vi "RTS Relay Status.vi"(0 "Chamber 1 Socket":string[][](array[string]), 1 "Tree Selection":T1="Select Room/Stall", 5 "Chamber 2 Socket":string[][](array[string]), 7 "Chamber 3 Socket":string[][](array[string]), 9 "Chamber 4 Socket":string[][](array[string]), 11 "error in (no error)":errorcluster, 12 "Extract Column":i32=73) -> (2 "Station 1":i32, 3 "Station 2":i32, 4 "Station 3":i32, 6 "Station 4":i32, 8 "Station 5":i32, 10 "Station 6":i32, 13 "Station 8":i32, 14 "Station 7":i32, 15 "error out":errorcluster)   [LabVIEW 2016]
uses:
  Type Definitions/RTS Room Selector.ctl
panel:
  in  "Debug":string[][](array[string])=[["System Date", "System Time", "Elapsed Time (sec)", "Elapsed Time (hrs)", "Voltage (V)", "RMS Current (Amps)", "Power (Watts)", "Watt Hours (Wh)", "Voltage Total Harmonic Distortion (%)", "Frequency (Hz)", "Apparent Power (VA)", "Power Factor", "TC 1", "TC 2", "TC 3", "TC 4", "TC 5", "TC 6", "TC 7", "TC 8", "TC 9", "TC 10", "TC 11", "TC 12", "TC 13", "TC 14", "TC 15", "TC 16", "TC 17", "TC 18", "TC 19", "TC 20", "TC 21", "TC 22", "TC 23", "TC 24", "TC 25", "TC 26", "TC 27", "TC 28", "TC 29", "TC 30", "AUX 1", "AUX 2", "CAL CL", "Room Setpoint Temperature", "Room Setpoint Humidity", "Room Temperature (°F)", "Room Humidity (%)", "Door Enable", "Room Setpoint Cool Temperature", "Room Setpoint Dehumidification Temperature", "Supply Temperature (°F)", "Cool Temperature (°F)", "Dehumidification Temperature (°F)", "Glycol Temperature (°F)", "Heat Rate (%)", "Steam Rate (%)", "Cool Rate (%)", "Dehumidification Rate (%)", "Room Status", "Room Dry P", "Room Dry I", "Room Humidity P", "Room Humidity I", "Room Heat P", "Room Heat I", "Room Cool Temperature P", "Room Cool Temperature I", "Room Dehumidification Temperature P", "Room Dehumidification Temperature I", "Voltage Setpoint 1", "60 Hz Power", "50 Hz Power", "120V Range", "240V Range", "Ground Line", "Ground Neutral", "Measure Ground Leakage Current", "Room OK", "S1 Freezer Relay", "S1 Cab Relay", "S1 Slide Relay", "Recording Data", "CVS Location", "Point Location"], ["01/23/2018", "08:26:39.773", "0.000000", "0.000000", "119.742401", "0.732354", "75.278603", "510.887438", "3.300000", "59.994091", "87.224380", "0.863045", "8.350000", "8.210000", "10.270000", "327.670000", "327.670000", "327.670000", "327.670000", "327.670000", "327.670000", "327.670000", "37.750000", "35.520000", "35.220000", "327.670000", "327.670000", "327.670000", "327.670000", "327.670000", "327.670000", "327.670000", "327.670000", "327.670000", "327.670000", "70.660000", "327.670000", "327.670000", "70.440000", "327.670000", "32767.000000", "32767.000000", "0.001000", "0.000000", "1.988000", "70.000000", "35.000000", "69.850000", "38.830000", "1.000000", "55.000000", "48.000000", "67.060000", "55.180000", "48.160000", "0.000000", "38.280000", "0.000000", "30.610000", "8.190000", "0.000000", "200.000000", "15000.000000", "400.000000", "15000.000000", "1000.000000", "2000.000000", "500.000000", "6000.000000", "500.000000", "6000.000000", "120.000000", "1.000000", "0.000000", "1.000000", "0.000000", "0", "1.000000", "0.000000", "0.000000", "0.000000", "0.000000", "0.000000", "FALSE", "", ""], ["System Date", "System Time", "Elapsed Time (sec)", "Elapsed Time (hrs)", "Voltage (V)", "RMS Current (Amps)", "Power (Watts)", "Watt Hours (Wh)", "Voltage Total Harmonic Distortion (%)", "Frequency (Hz)", "Apparent Power (VA)", "Power Factor", "TC 1", "TC 2", "TC 3", "TC 4", "TC 5", "TC 6", "TC 7", "TC 8", "TC 9", "TC 10", "TC 11", "TC 12", "TC 13", "TC 14", "TC 15", "TC 16", "TC 17", "TC 18", "TC 19", "TC 20", "TC 21", "TC 22", "TC 23", "TC 24", "TC 25", "TC 26", "TC 27", "TC 28", "TC 29", "TC 30", "AUX 1", "AUX 2", "CAL CL", "Room Setpoint Temperature", "Room Setpoint Humidity", "Room Temperature (°F)", "Room Humidity (%)", "Door Enable", "Room Setpoint Cool Temperature", "Room Setpoint Dehumidification Temperature", "Supply Temperature (°F)", "Cool Temperature (°F)", "Dehumidification Temperature (°F)", "Glycol Temperature (°F)", "Heat Rate (%)", "Steam Rate (%)", "Cool Rate (%)", "Dehumidification Rate (%)", "Room Status", "Room Dry P", "Room Dry I", "Room Humidity P", "Room Humidity I", "Room Heat P", "Room Heat I", "Room Cool Temperature P", "Room Cool Temperature I", "Room Dehumidification Temperature P", "Room Dehumidification Temperature I", "Voltage Setpoint 2", "60 Hz Power", "50 Hz Power", "120V Range", "240V Range", "Ground Line", "Ground Neutral", "Measure Ground Leakage Current", "Fault", "S2 Freezer Relay", "S2 Cab Relay", "S2 Slide Relay", "Recording Data", "CVS Location", "Point Location"], ["01/23/2018", "08:26:39.773", "0.000000", "0.000000", "114.834923", "0.030745", "0.141378", "25815.620693", "3.200000", "59.993526", "3.530576", "1.000000", "4.260000", "4.640000", "5.190000", "327.670000", "327.670000", "327.670000", "327.670000", "327.670000", "327.670000", "327.670000", "38.960000", "40.520000", "41.760000", "327.670000", "327.670000", "327.670000", "327.670000", "327.670000", "327.670000", "327.670000", "327.670000", "327.670000", "327.670000", "70.050000", "327.670000", "327.670000", "70.140000", "327.670000", "32767.000000", "32767.000000", "0.000000", "0.000000", "1.990000", "70.000000", "35.000000", "69.850000", "38.830000", "1.000000", "55.000000", "48.000000", "67.060000", "55.180000", "48.160000", "0.000000", "38.280000", "0.000000", "30.610000", "8.190000", "0.000000", "200.000000", "15000.000000", "400.000000", "15000.000000", "1000.000000", "2000.000000", "500.000000", "6000.000000", "500.000000", "6000.000000", "115.000000", "1.000000", "0.000000", "1.000000", "0.000000", "0", "1.000000", "0.000000", "0.000000", "0.000000", "0.000000", "0.000000", "FALSE", "", ""], ["System Date", "System Time", "Elapsed Time (sec)", "Elapsed Time (hrs)", "Voltage (V)", "RMS Current (Amps)", "Power (Watts)", "Watt Hours (Wh)", "Voltage Total Harmonic Distortion (%)", "Frequency (Hz)", "Apparent Power (VA)", "Power Factor", "TC 1", "TC 2", "TC 3", "TC 4", "TC 5", "TC 6", "TC 7", "TC 8", "TC 9", "TC 10", "TC 11", "TC 12", "TC 13", "TC 14", "TC 15", "TC 16", "TC 17", "TC 18", "TC 19", "TC 20", "TC 21", "TC 22", "TC 23", "TC 24", "TC 25", "TC 26", "TC 27", "TC 28", "TC 29", "TC 30", "AUX 1", "AUX 2", "CAL CL", "Room Setpoint Temperature", "Room Setpoint Humidity", "Room Temperature (°F)", "Room Humidity (%)", "Door Enable", "Room Setpoint Cool Temperature", "Room Setpoint Dehumidification Temperature", "Supply Temperature (°F)", "Cool Temperature (°F)", "Dehumidification Temperature (°F)", "Glycol Temperature (°F)", "Heat Rate (%)", "Steam Rate (%)", "Cool Rate (%)", "Dehumidification Rate (%)", "Room Status", "Room Dry P", "Room Dry I", "Room Humidity P", "Room Humidity I", "Room Heat P", "Room Heat I", "Room Cool Temperature P", "Room Cool Temperature I", "Room Dehumidification Temperature P", "Room Dehumidification Temperature I", "Voltage Setpoint 3", "60 Hz Power", "50 Hz Power", "120V Range", "240V Range", "Ground Line", "Ground Neutral", "Measure Ground Leakage Current", "Room Heat", "S3 Freezer Relay", "S3 Cab Relay", "S3 Slide Relay", "Recording Data", "CVS Location", "Point Location"], ["01/23/2018", "08:26:39.773", "0.000000", "0.000000", "114.806053", "0.030078", "0.138114", "27523.299150", "3.300000", "59.994259", "3.453151", "1.000000", "0.550000", "0.550000", "1.570000", "327.670000", "327.670000", "327.670000", "327.670000", "327.670000", "327.670000", "327.670000", "37.750000", "38.130000", "38.080000", "327.670000", "327.670000", "327.670000", "327.670000", "327.670000", "327.670000", "327.670000", "327.670000", "327.670000", "327.670000", "70.140000", "327.670000", "327.670000", "70.300000", "327.670000", "32767.000000", "32767.000000", "0.001000", "0.000000", "1.963000", "70.000000", "35.000000", "69.850000", "38.830000", "1.000000", "55.000000", "48.000000", "67.060000", "55.180000", "48.160000", "0.000000", "38.280000", "0.000000", "30.610000", "8.190000", "0.000000", "200.000000", "15000.000000", "400.000000", "15000.000000", "1000.000000", "2000.000000", "500.000000", "6000.000000", "500.000000", "6000.000000", "115.000000", "1.000000", "0.000000", "1.000000", "0.000000", "0", "1.000000", "1.000000", "0.000000", "0.000000", "0.000000", "0.000000", "FALSE", "", ""], ["System Date", "System Time", "Elapsed Time (sec)", "Elapsed Time (hrs)", "Voltage (V)", "RMS Current (Amps)", "Power (Watts)", "Watt Hours (Wh)", "Voltage Total Harmonic Distortion (%)", "Frequency (Hz)", "Apparent Power (VA)", "Power Factor", "TC 1", "TC 2", "TC 3", "TC 4", "TC 5", "TC 6", "TC 7", "TC 8", "TC 9", "TC 10", "TC 11", "TC 12", "TC 13", "TC 14", "TC 15", "TC 16", "TC 17", "TC 18", "TC 19", "TC 20", "TC 21", "TC 22", "TC 23", "TC 24", "TC 25", "TC 26", "TC 27", "TC 28", "TC 29", "TC 30", "AUX 1", "AUX 2", "CAL CL", "Room Setpoint Temperature", "Room Setpoint Humidity", "Room Temperature (°F)", "Room Humidity (%)", "Door Enable", "Room Setpoint Cool Temperature", "Room Setpoint Dehumidification Temperature", "Supply Temperature (°F)", "Cool Temperature (°F)", "Dehumidification Temperature (°F)", "Glycol Temperature (°F)", "Heat Rate (%)", "Steam Rate (%)", "Cool Rate (%)", "Dehumidification Rate (%)", "Room Status", "Room Dry P", "Room Dry I", "Room Humidity P", "Room Humidity I", "Room Heat P", "Room Heat I", "Room Cool Temperature P", "Room Cool Temperature I", "Room Dehumidification Temperature P", "Room Dehumidification Temperature I", "Voltage Setpoint 4", "60 Hz Power", "50 Hz Power", "120V Range", "240V Range", "Ground Line", "Ground Neutral", "Measure Ground Leakage Current", "Room Blower", "S4 Freezer Relay", "S4 Cab Relay", "S4 Slide Relay", "Recording Data", "CVS Location", "Point Location"], ["01/23/2018", "08:26:39.774", "0.000000", "0.000000", "115.383408", "0.030500", "0.137436", "25916.370885", "3.200000", "59.993530", "3.519194", "1.000000", "8.980000", "7.010000", "6.290000", "327.670000", "327.670000", "327.670000", "327.670000", "327.670000", "327.670000", "327.670000", "41.400000", "41.400000", "41.810000", "327.670000", "327.670000", "327.670000", "327.670000", "327.670000", "327.670000", "327.670000", "327.670000", "327.670000", "327.670000", "70.630000", "327.670000", "327.670000", "70.930000", "327.670000", "32767.000000", "32767.000000", "0.001000", "0.001000", "2.005000", "70.000000", "35.000000", "69.850000", "38.830000", "1.000000", "55.000000", "48.000000", "67.060000", "55.180000", "48.160000", "0.000000", "38.280000", "0.000000", "30.610000", "8.190000", "0.000000", "200.000000", "15000.000000", "400.000000", "15000.000000", "1000.000000", "2000.000000", "500.000000", "6000.000000", "500.000000", "6000.000000", "115.000000", "1.000000", "0.000000", "1.000000", "0.000000", "0", "1.000000", "1.000000", "0.000000", "0.000000", "0.000000", "0.000000", "FALSE", "", ""], ["System Date", "System Time", "Elapsed Time (sec)", "Elapsed Time (hrs)", "Voltage (V)", "RMS Current (Amps)", "Power (Watts)", "Watt Hours (Wh)", "Voltage Total Harmonic Distortion (%)", "Frequency (Hz)", "Apparent Power (VA)", "Power Factor", "TC 1", "TC 2", "TC 3", "TC 4", "TC 5", "TC 6", "TC 7", "TC 8", "TC 9", "TC 10", "TC 11", "TC 12", "TC 13", "TC 14", "TC 15", "TC 16", "TC 17", "TC 18", "TC 19", "TC 20", "TC 21", "TC 22", "TC 23", "TC 24", "TC 25", "TC 26", "TC 27", "TC 28", "TC 29", "TC 30", "AUX 1", "AUX 2", "CAL CL", "Room Setpoint Temperature", "Room Setpoint Humidity", "Room Temperature (°F)", "Room Humidity (%)", "Door Enable", "Room Setpoint Cool Temperature", "Room Setpoint Dehumidification Temperature", "Supply Temperature (°F)", "Cool Temperature (°F)", "Dehumidification Temperature (°F)", "Glycol Temperature (°F)", "Heat Rate (%)", "Steam Rate (%)", "Cool Rate (%)", "Dehumidification Rate (%)", "Room Status", "Room Dry P", "Room Dry I", "Room Humidity P", "Room Humidity I", "Room Heat P", "Room Heat I", "Room Cool Temperature P", "Room Cool Temperature I", "Room Dehumidification Temperature P", "Room Dehumidification Temperature I", "Voltage Setpoint 5", "60 Hz Power", "50 Hz Power", "120V Range", "240V Range", "Ground Line", "Ground Neutral", "Measure Ground Leakage Current", "Spare", "S5 Freezer Relay", "S5 Cab Relay", "S5 Slide Relay", "Recording Data", "CVS Location", "Point Location"], ["01/23/2018", "08:26:39.774", "0.000000", "0.000000", "114.998505", "0.000000", "0.000000", "0.000000", "3.200000", "59.993629", "0.000000", "1.000000", "327.670000", "327.670000", "70.220000", "327.670000", "327.670000", "327.670000", "327.670000", "327.670000", "327.670000", "327.670000", "70.410000", "70.140000", "70.080000", "327.670000", "327.670000", "327.670000", "327.670000", "327.670000", "327.670000", "327.670000", "327.670000", "327.670000", "327.670000", "69.780000", "327.670000", "327.670000", "327.670000", "327.670000", "32767.000000", "32767.000000", "0.000000", "0.001000", "1.998000", "70.000000", "35.000000", "69.850000", "38.830000", "1.000000", "55.000000", "48.000000", "67.060000", "55.180000", "48.160000", "0.000000", "38.280000", "0.000000", "30.610000", "8.190000", "0.000000", "200.000000", "15000.000000", "400.000000", "15000.000000", "1000.000000", "2000.000000", "500.000000", "6000.000000", "500.000000", "6000.000000", "115.000000", "1.000000", "0.000000", "1.000000", "0.000000", "0", "1.000000", "0.000000", "0.000000", "0.000000", "0.000000", "0.000000", "FALSE", "", ""], ["System Date", "System Time", "Elapsed Time (sec)", "Elapsed Time (hrs)", "Voltage (V)", "RMS Current (Amps)", "Power (Watts)", "Watt Hours (Wh)", "Voltage Total Harmonic Distortion (%)", "Frequency (Hz)", "Apparent Power (VA)", "Power Factor", "TC 1", "TC 2", "TC 3", "TC 4", "TC 5", "TC 6", "TC 7", "TC 8", "TC 9", "TC 10", "TC 11", "TC 12", "TC 13", "TC 14", "TC 15", "TC 16", "TC 17", "TC 18", "TC 19", "TC 20", "TC 21", "TC 22", "TC 23", "TC 24", "TC 25", "TC 26", "TC 27", "TC 28", "TC 29", "TC 30", "AUX 1", "AUX 2", "CAL CL", "Room Setpoint Temperature", "Room Setpoint Humidity", "Room Temperature (°F)", "Room Humidity (%)", "Door Enable", "Room Setpoint Cool Temperature", "Room Setpoint Dehumidification Temperature", "Supply Temperature (°F)", "Cool Temperature (°F)", "Dehumidification Temperature (°F)", "Glycol Temperature (°F)", "Heat Rate (%)", "Steam Rate (%)", "Cool Rate (%)", "Dehumidification Rate (%)", "Room Status", "Room Dry P", "Room Dry I", "Room Humidity P", "Room Humidity I", "Room Heat P", "Room Heat I", "Room Cool Temperature P", "Room Cool Temperature I", "Room Dehumidification Temperature P", "Room Dehumidification Temperature I", "Voltage Setpoint 6", "60 Hz Power", "50 Hz Power", "120V Range", "240V Range", "Ground Line", "Ground Neutral", "Measure Ground Leakage Current", "Room Pump", "S6 Freezer Relay", "S6 Cab Relay", "S6 Slide Relay", "Recording Data", "CVS Location", "Point Location"], ["01/23/2018", "08:26:39.774", "0.000000", "0.000000", "114.796432", "0.000000", "0.000000", "0.000000", "3.600000", "59.994347", "0.000000", "1.000000", "327.670000", "327.670000", "327.670000", "327.670000", "327.670000", "327.670000", "327.670000", "327.670000", "327.670000", "327.670000", "327.670000", "327.670000", "327.670000", "327.670000", "327.670000", "327.670000", "327.670000", "327.670000", "327.670000", "327.670000", "327.670000", "327.670000", "327.670000", "327.670000", "327.670000", "327.670000", "327.670000", "327.670000", "32767.000000", "32767.000000", "0.001000", "0.000000", "1.995000", "70.000000", "35.000000", "69.850000", "38.830000", "1.000000", "55.000000", "48.000000", "67.060000", "55.180000", "48.160000", "0.000000", "38.280000", "0.000000", "30.610000", "8.190000", "0.000000", "200.000000", "15000.000000", "400.000000", "15000.000000", "1000.000000", "2000.000000", "500.000000", "6000.000000", "500.000000", "6000.000000", "115.000000", "1.000000", "0.000000", "1.000000", "0.000000", "0", "1.000000", "1.000000", "0.000000", "0.000000", "0.000000", "0.000000", "FALSE", "", ""], ["System Date", "System Time", "Elapsed Time (sec)", "Elapsed Time (hrs)", "Voltage (V)", "RMS Current (Amps)", "Power (Watts)", "Watt Hours (Wh)", "Voltage Total Harmonic Distortion (%)", "Frequency (Hz)", "Apparent Power (VA)", "Power Factor", "TC 1", "TC 2", "TC 3", "TC 4", "TC 5", "TC 6", "TC 7", "TC 8", "TC 9", "TC 10", "TC 11", "TC 12", "TC 13", "TC 14", "TC 15", "TC 16", "TC 17", "TC 18", "TC 19", "TC 20", "TC 21", "TC 22", "TC 23", "TC 24", "TC 25", "TC 26", "TC 27", "TC 28", "TC 29", "TC 30", "AUX 1", "AUX 2", "CAL CL", "Room Setpoint Temperature", "Room Setpoint Humidity", "Room Temperature (°F)", "Room Humidity (%)", "Door Enable", "Room Setpoint Cool Temperature", "Room Setpoint Dehumidification Temperature", "Supply Temperature (°F)", "Cool Temperature (°F)", "Dehumidification Temperature (°F)", "Glycol Temperature (°F)", "Heat Rate (%)", "Steam Rate (%)", "Cool Rate (%)", "Dehumidification Rate (%)", "Room Status", "Room Dry P", "Room Dry I", "Room Humidity P", "Room Humidity I", "Room Heat P", "Room Heat I", "Room Cool Temperature P", "Room Cool Temperature I", "Room Dehumidification Temperature P", "Room Dehumidification Temperature I", "Voltage Setpoint 7", "60 Hz Power", "50 Hz Power", "120V Range", "240V Range", "Ground Line", "Ground Neutral", "Measure Ground Leakage Current", "Spare", "S7 Freezer Relay", "S7 Cab Relay", "S7 Slide Relay", "Recording Data", "CVS Location", "Point Location"], ["01/23/2018", "08:26:39.774", "0.000000", "0.000000", "115.017746", "0.000000", "0.000000", "0.000000", "3.500000", "59.993889", "0.000000", "1.000000", "70.660000", "70.710000", "70.710000", "327.670000", "327.670000", "327.670000", "327.670000", "327.670000", "327.670000", "327.670000", "327.670000", "70.520000", "70.520000", "327.670000", "327.670000", "327.670000", "327.670000", "327.670000", "327.670000", "327.670000", "327.670000", "327.670000", "327.670000", "327.670000", "327.670000", "327.670000", "327.670000", "327.670000", "32767.000000", "32767.000000", "0.000000", "0.000000", "2.003000", "70.000000", "35.000000", "69.850000", "38.830000", "1.000000", "55.000000", "48.000000", "67.060000", "55.180000", "48.160000", "0.000000", "38.280000", "0.000000", "30.610000", "8.190000", "0.000000", "200.000000", "15000.000000", "400.000000", "15000.000000", "1000.000000", "2000.000000", "500.000000", "6000.000000", "500.000000", "6000.000000", "115.000000", "1.000000", "0.000000", "1.000000", "0.000000", "0", "1.000000", "0.000000", "0.000000", "0.000000", "0.000000", "0.000000", "FALSE", "", ""], ["System Date", "System Time", "Elapsed Time (sec)", "Elapsed Time (hrs)", "Voltage (V)", "RMS Current (Amps)", "Power (Watts)", "Watt Hours (Wh)", "Voltage Total Harmonic Distortion (%)", "Frequency (Hz)", "Apparent Power (VA)", "Power Factor", "TC 1", "TC 2", "TC 3", "TC 4", "TC 5", "TC 6", "TC 7", "TC 8", "TC 9", "TC 10", "TC 11", "TC 12", "TC 13", "TC 14", "TC 15", "TC 16", "TC 17", "TC 18", "TC 19", "TC 20", "TC 21", "TC 22", "TC 23", "TC 24", "TC 25", "TC 26", "TC 27", "TC 28", "TC 29", "TC 30", "AUX 1", "AUX 2", "CAL CL", "Room Setpoint Temperature", "Room Setpoint Humidity", "Room Temperature (°F)", "Room Humidity (%)", "Door Enable", "Room Setpoint Cool Temperature", "Room Setpoint Dehumidification Temperature", "Supply Temperature (°F)", "Cool Temperature (°F)", "Dehumidification Temperature (°F)", "Glycol Temperature (°F)", "Heat Rate (%)", "Steam Rate (%)", "Cool Rate (%)", "Dehumidification Rate (%)", "Room Status", "Room Dry P", "Room Dry I", "Room Humidity P", "Room Humidity I", "Room Heat P", "Room Heat I", "Room Cool Temperature P", "Room Cool Temperature I", "Room Dehumidification Temperature P", "Room Dehumidification Temperature I", "Voltage Setpoint 8", "60 Hz Power", "50 Hz Power", "120V Range", "240V Range", "Ground Line", "Ground Neutral", "Measure Ground Leakage Current", "Spare", "S8 Freezer Relay", "S8 Cab Relay", "S8 Slide Relay", "Recording Data", "CVS Location", "Point Location"], ["01/23/2018", "08:26:39.774", "0.000000", "0.000000", "115.219826", "0.000000", "0.000000", "0.000000", "3.600000", "59.993702", "0.000000", "1.000000", "70.630000", "70.520000", "70.630000", "327.670000", "327.670000", "327.670000", "327.670000", "327.670000", "327.670000", "327.670000", "70.770000", "70.440000", "70.410000", "327.670000", "327.670000", "327.670000", "327.670000", "327.670000", "327.670000", "327.670000", "327.670000", "327.670000", "327.670000", "327.670000", "327.670000", "327.670000", "327.670000", "327.670000", "32767.000000", "32767.000000", "0.000000", "0.000000", "1.955000", "70.000000", "35.000000", "69.850000", "38.830000", "1.000000", "55.000000", "48.000000", "67.060000", "55.180000", "48.160000", "0.000000", "38.280000", "0.000000", "30.610000", "8.190000", "0.000000", "200.000000", "15000.000000", "400.000000", "15000.000000", "1000.000000", "2000.000000", "500.000000", "6000.000000", "500.000000", "6000.000000", "115.000000", "1.000000", "0.000000", "1.000000", "0.000000", "1", "1.000000", "0.000000", "0.000000", "0.000000", "0.000000", "1.000000", "FALSE", "", ""]]
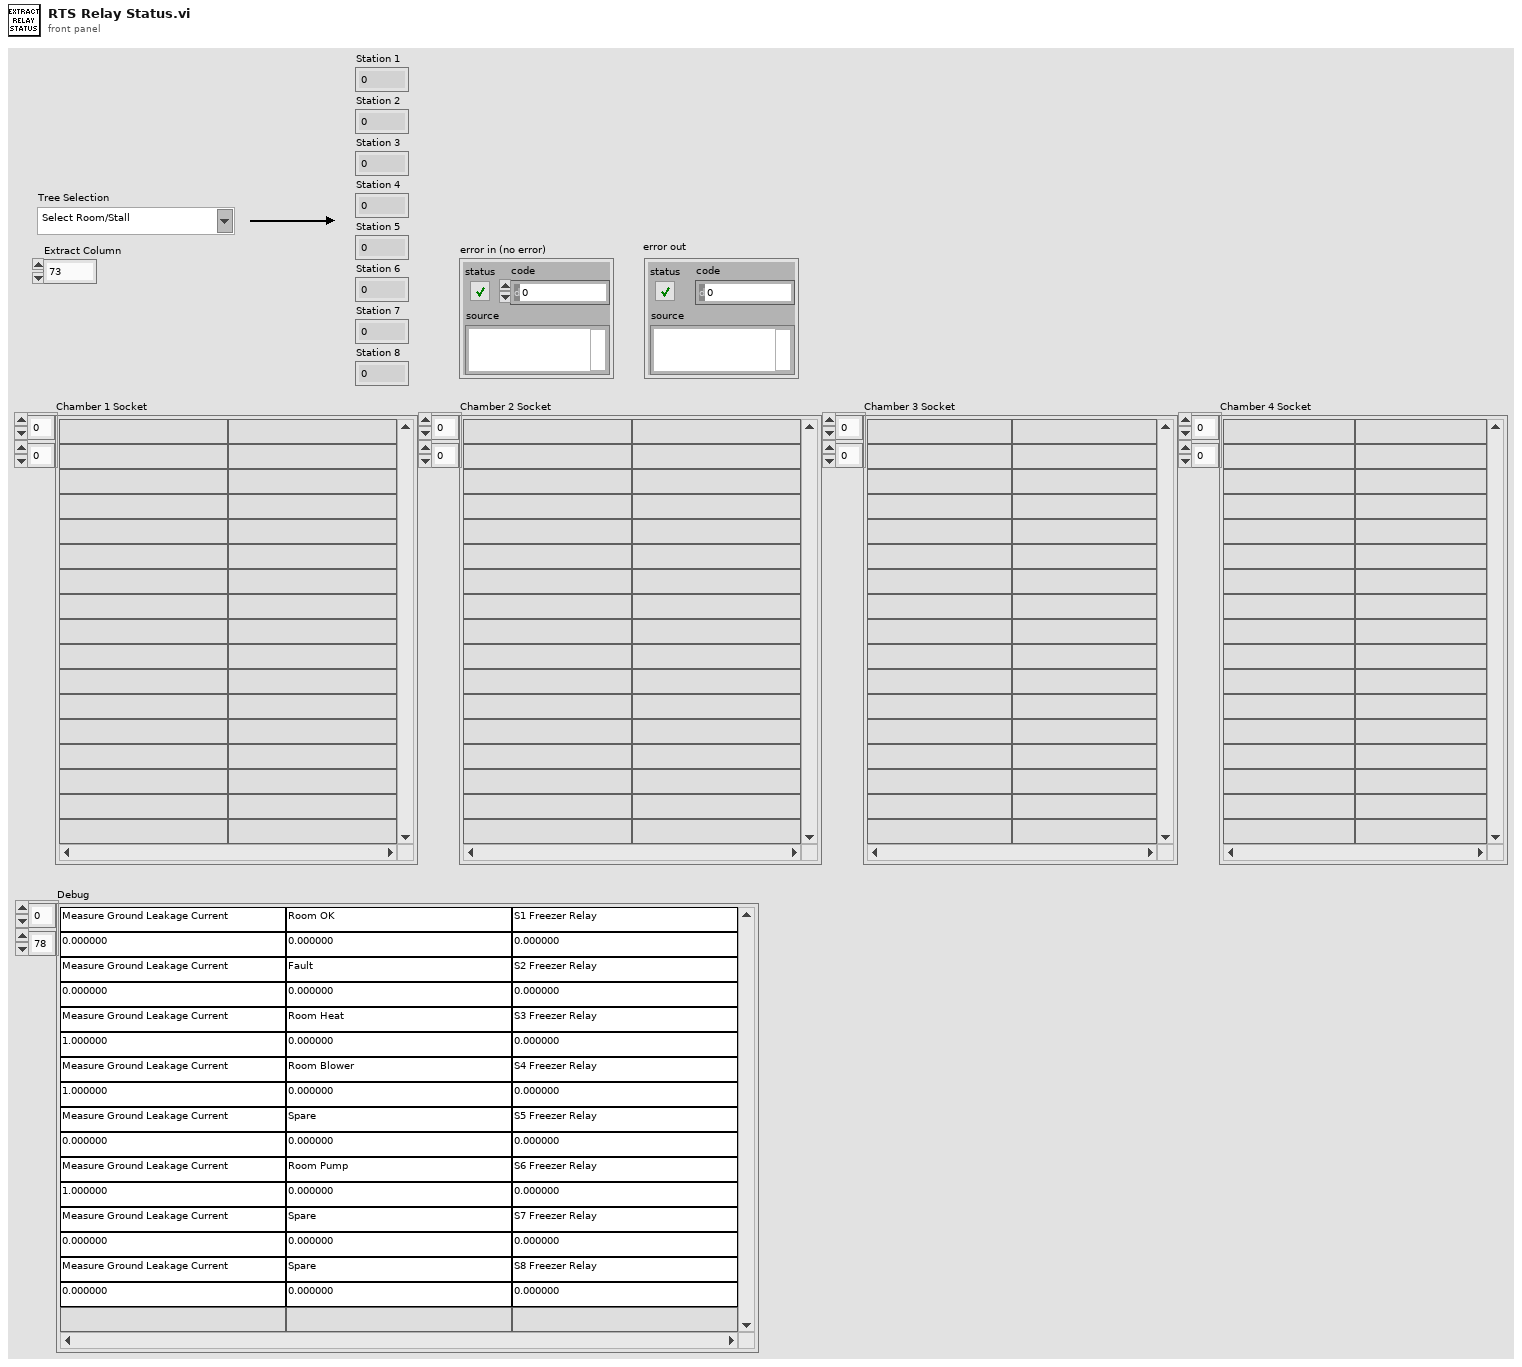
[diagram p1: front panel]
types:
  T1 = typedef "RTS Room Selector.ctl" = string
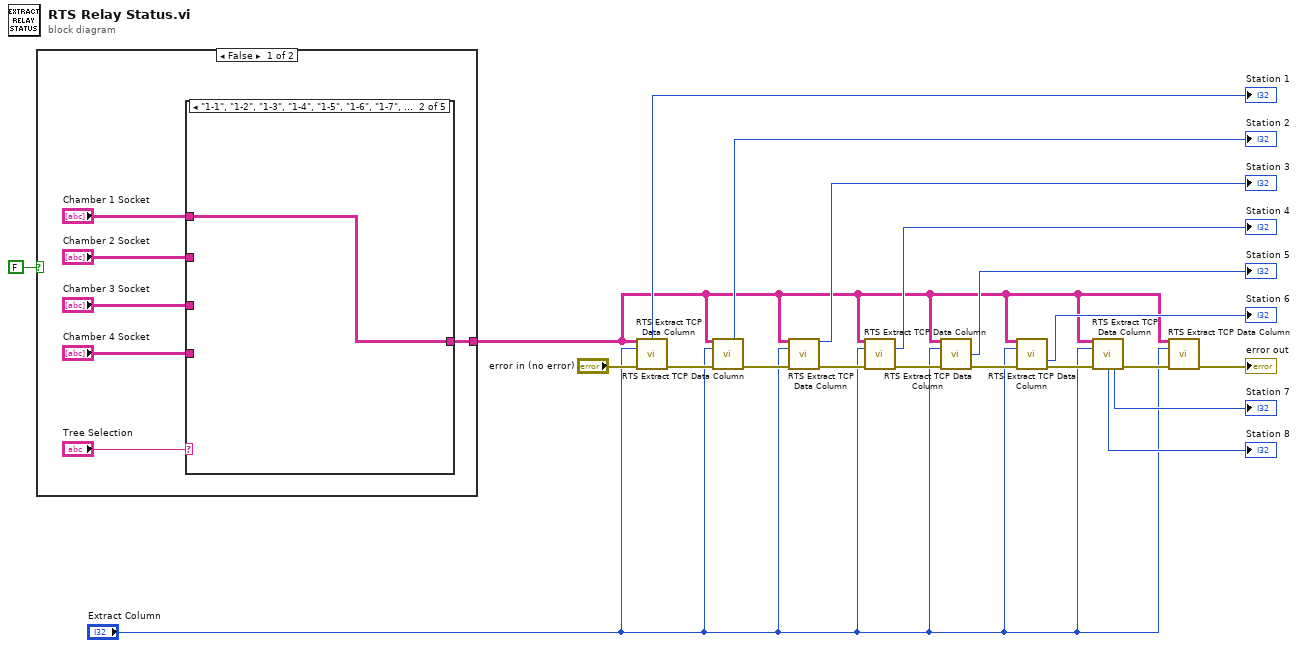
[diagram p0: block diagram]
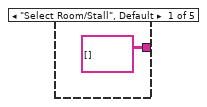
[diagram p2: hidden frame]
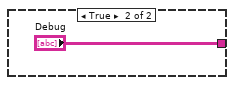
[diagram p6: hidden frame]
diagram:
  n1 = case shown="False" FALSE {
    tunnel: [w21 "Debug"] -> w1
    frame False {
      n2 = case shown="\"1-1\", \"1-2\", \"1-3\", \"1-4\", \"1-5\", \"1-6\", \"1-7\", \"1-8\"" "Tree Selection" {
        tunnel: "Chamber 1 Socket" -> [_ w28 _ _ _]
        tunnel: [string[][] [] ("Chamber 4 Socket") w28 w29 w30 w31] -> w21
        tunnel: "Chamber 2 Socket" -> [_ _ w29 _ _]
        tunnel: "Chamber 3 Socket" -> [_ _ _ w30 _]
        tunnel: "Chamber 4 Socket" -> [_ _ _ _ w31]
        frame "Select Room/Stall", Default {
        }
        frame "1-1", "1-2", "1-3", "1-4", "1-5", "1-6", "1-7", "1-8" {
        }
        frame "2-1", "2-2", "2-3", "2-4", "2-5", "2-6", "2-7", "2-8" {
        }
        frame "3-1", "3-2", "3-3", "3-4", "3-5", "3-6", "3-7", "3-8" {
        }
        frame "4-1", "4-2", "4-3", "4-4", "4-5", "4-6", "4-7", "4-8" {
        }
      }
    }
    frame True {
    }
  }
  n3 = call "RTS Extract TCP Data Column.vi"("Chamber 1 Socket"=w1, "Extract Column"="Extract Column", "Error In"="error in (no error)") -> ("Station 1"=→"Station 1":i32, "Error Out"=w4:errorcluster)  [unwired: 4 in, 7 out]
  n4 = call "RTS Extract TCP Data Column.vi"("Chamber 1 Socket"=w1, "Extract Column"="Extract Column", "Error In"=w4) -> ("Station 2"=→"Station 2":i32, "Error Out"=w5:errorcluster)  [unwired: 4 in, 7 out]
  n5 = call "RTS Extract TCP Data Column.vi"("Chamber 1 Socket"=w1, "Extract Column"="Extract Column", "Error In"=w5) -> ("Station 3"=→"Station 3":i32, "Error Out"=w6:errorcluster)  [unwired: 4 in, 7 out]
  n6 = call "RTS Extract TCP Data Column.vi"("Chamber 1 Socket"=w1, "Extract Column"="Extract Column", "Error In"=w6) -> ("Station 4"=→"Station 4":i32, "Error Out"=w10:errorcluster)  [unwired: 4 in, 7 out]
  n7 = call "RTS Extract TCP Data Column.vi"("Chamber 1 Socket"=w1, "Extract Column"="Extract Column", "Error In"=w10) -> ("Station 5"=→"Station 5":i32, "Error Out"=w9:errorcluster)  [unwired: 4 in, 7 out]
  n8 = call "RTS Extract TCP Data Column.vi"("Chamber 1 Socket"=w1, "Extract Column"="Extract Column", "Error In"=w9) -> ("Station 6"=→"Station 6":i32, "Error Out"=w8:errorcluster)  [unwired: 4 in, 7 out]
  n9 = call "RTS Extract TCP Data Column.vi"("Chamber 1 Socket"=w1, "Extract Column"="Extract Column", "Error In"=w8) -> ("Station 8"=→"Station 8":i32, "Station 7"=→"Station 7":i32, "Error Out"=w7:errorcluster)  [unwired: 4 in, 6 out]
  n10 = call "RTS Extract TCP Data Column.vi"("Chamber 1 Socket"=w1, "Extract Column"="Extract Column", "Error In"=w7) -> ("Error Out"=→"error out":errorcluster)  [unwired: 4 in, 8 out]
